vi "write file header Gamry v3.vi"(4 "Chamber pressure (MPa)":dbl=0.1, 5 "Chamber temp (K)":dbl, 6 "error in":errorcluster, 7 "Description":string, 8 "testp":T1={"Start F"=20.0, "Stop F"=1000.0, "# Steps"=200, "Init Z Guess"=100.0, "Device #"=1, "Vamp (V)"=10.0} caption="Test Parameters" {"Vamp (V)" min=0.0001 max=10; "Device #" min=0 max=10 step=1; "Init Z Guess" format="%_6g"; "# Steps" min=1 max=1800 step=1; "Stop F" min=0.001 max=2000000 step=1 format="%^#_3e"; "Start F" min=0.001 max=2000000 step=1 format="%^#_3e"}, 9 "Output refnum":refnum<file>) -> (0 "error out":errorcluster, 2 "Refnum out":refnum<file>)   [LabVIEW 2018]
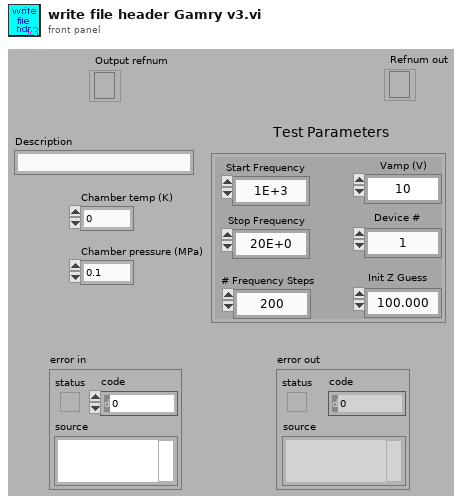
[diagram p1: front panel]
types:
  T1 = cluster{"Start F":sgl, "Stop F":sgl, "# Steps":u32, "Init Z Guess":sgl, "Device #":i16, "Vamp (V)":sgl}
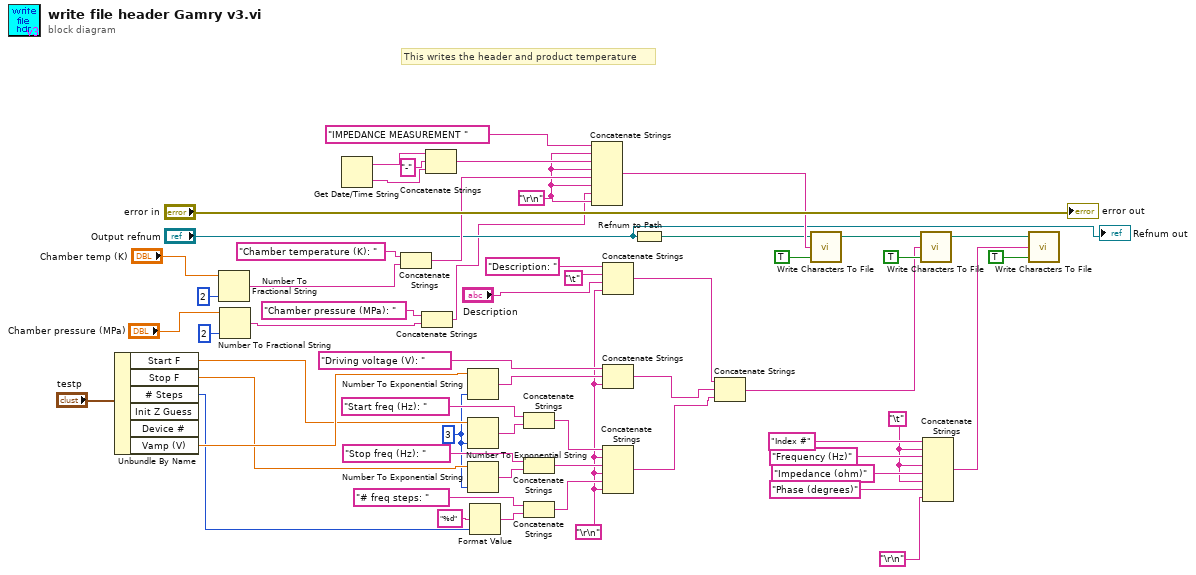
[diagram p0: block diagram]
diagram:
  w11 = 3
  w3 = "\r\n"
  w9 = "\r\n"
  w38 = "\t"
  # "This writes the header and product temperature"
  n1 = Unbundle By Name("testp") -> ("Start F"=w20:sgl, "Stop F"=w19:sgl, "# Steps"=w14:u32, "Vamp (V)"=w21:sgl)  [unwired: 2 out]
  n2 = Number To Fractional String(number="Chamber temp (K)", precision (6)=i16 2) -> (F-format string=w31:string)  [unwired: 2 in]
  n3 = Number To Fractional String(number="Chamber pressure (MPa)", precision (6)=i16 2) -> (F-format string=w4:string)  [unwired: 2 in]
  n4 = Get Date/Time String() -> (date string=w33:string, time string=w32:string)  [unwired: 3 in]
  n5 = Concatenate Strings("Chamber temperature (K): " ("string"), w31) -> (w17:string)
  n6 = Concatenate Strings("Chamber pressure (MPa): " ("string"), w4) -> (w2:string)
  n7 = Concatenate Strings(w33, "-" ("string"), w32) -> (w25:string)
  n8 = Number To Exponential String(number=w21, precision (6)=w11) -> (E-format string=w40:string)  [unwired: 2 in]
  n9 = Number To Exponential String(number=w20, precision (6)=w11) -> (E-format string=w50:string)  [unwired: 2 in]
  n10 = Number To Exponential String(number=w19, precision (6)=w11) -> (E-format string=w49:string)  [unwired: 2 in]
  n11 = Format Value(format string="%d", value (0)=w14) -> (output string=w12:string)  [unwired: 1 in]
  n12 = Concatenate Strings("Start freq (Hz): " ("string"), w50) -> (w48:string)
  n13 = Concatenate Strings("Stop freq (Hz): " ("string"), w49) -> (w47:string)
  n14 = Concatenate Strings("# freq steps: " ("string"), w12) -> (w46:string)
  n15 = Concatenate Strings("IMPEDANCE MEASUREMENT " ("string"), w3, w25, w3, w17, w3, w2, w3) -> (w24:string)
  n16 = Concatenate Strings("Description: " ("string"), "\t", "Description", w9) -> (w18:string)
  n17 = Concatenate Strings("Driving voltage (V): " ("string"), w40, w9) -> (w16:string)
  n18 = Concatenate Strings(w48, w9, w47, w9, w46, w9) -> (w15:string)
  n19 = Refnum to Path(1:"Output refnum") -> (0:w8:path)
  n20 = Concatenate Strings(w18, w16, w15) -> (w28:string)
  n21 = call <vilib>:"Write Characters To File.vi"("append to file? (new file:F)"=TRUE, "character string"=w24, "file path (dialog if empty)"=w8) -> ("new file path (Not A Path if cancelled)"=w45:path)  [unwired: 2 in]
  n22 = call <vilib>:"Write Characters To File.vi"("append to file? (new file:F)"=TRUE, "character string"=w28, "file path (dialog if empty)"=w45) -> ("new file path (Not A Path if cancelled)"=w56:path)  [unwired: 2 in]
  n23 = Concatenate Strings("Index #", w38, "Frequency (Hz)", w38, "Impedance (ohm)", w38, "Phase (degrees)", "\r\n") -> (w41:string)
  n24 = call <vilib>:"Write Characters To File.vi"("append to file? (new file:F)"=TRUE, "character string"=w41, "file path (dialog if empty)"=w56) -> ()  [unwired: 2 in, 1 out]
  "error out" <- "error in"
  "Refnum out" <- "Output refnum"
